vi "Reload Bitfile.vi"(8 "error in (no error)":errorcluster, 10 "RIO Addresses (all)":string[](array[string]), 11 "Node Ptr":u64) -> (0 "error out":errorcluster, 3 "Node Ptr out":T1=18446744073709551615 format="%.0x")   [LabVIEW 2015, in "Engine Simulation Toolkit System Explorer.lvlib"]
uses:
  Engine Simulation Toolkit System Explorer.lvlib
  <vilib>/NI Veristand/Custom Device API/Custom Device Item Ref.ctl
  Shared/Properties.vi
  <vilib>/NI Veristand/Custom Device API/Get Item Property (String Array).vi
  <vilib>/NI Veristand/Custom Device API/Get Item Property (Dependent File).vi
  <vilib>/NI VeriStand/Custom Device API/Custom Device API.lvlib
  Shared/Engine Simulation Toolkit Shared.lvlib
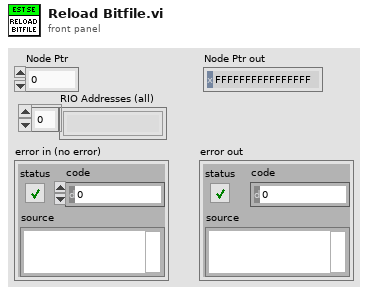
[diagram p1: front panel]
types:
  T1 = typedef "Custom Device API.lvlib/Custom Device Item Ref.ctl" = u64
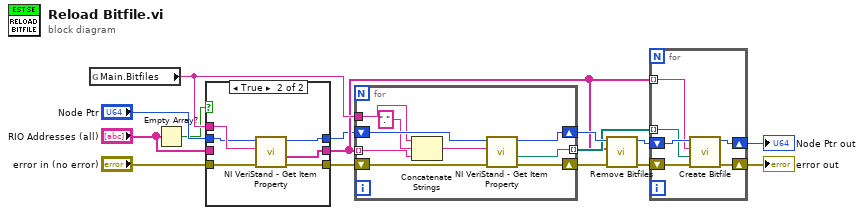
[diagram p0: block diagram]
diagram:
  n1 = global read "Properties.vi" "Main.Bitfiles"() -> (w15:string)
  n2 = Empty Array?(array="RIO Addresses (all)") -> (empty?=w2:bool)
  n3 = case shown="True" w2 {
    tunnel: w15 -> [_ w24]
    tunnel: [w18 w23] -> w11
    tunnel: [w17 w22] -> w10
    tunnel: [w16 w21] -> w9
    tunnel: "error in (no error)" -> [w17 w20]
    tunnel: "Node Ptr" -> [w16 w19]
    tunnel: "RIO Addresses (all)" -> [w18 _]
    frame False {
    }
    frame True {
      n4 = call-poly <vilib>:"NI VeriStand - Get Item Property.vi"("error in (no error)"=w20, "Property Name"=w24, "Item Ref in"=w19) -> ("error out"=w22:errorcluster, "Value"=w23:string[], "Item Ref out"=w21:T1)  [unwired: 5 in, 1 out]
    }
  }
  n5 = for {
    shift-right: [w30] -> w14
    shift-left: w9 -> [w33]
    shift-right: [w31] -> w13
    shift-left: w10 -> [w32]
    tunnel: w11 -> [w28] mode=indexing
    tunnel: [w26] -> w12 mode=indexing
    tunnel: w15 -> [w25]
    n6 = Concatenate Strings(w25, "." ("string"), w28) -> (w27:string)
    n7 = call-poly <vilib>:"NI VeriStand - Get Item Property.vi"("error in (no error)"=w32, "Property Name"=w27, "Item Ref in"=w33) -> ("error out"=w31:errorcluster, "Path"=w26:path, "Item Ref out"=w30:T1)  [unwired: 4 in, 2 out]
  }
  n8 = call "Remove Bitfiles.vi"("error in (no error)"=w13, "RIO Addresses"=w11, "Item Ref in"=w14) -> ("error out"=w4:errorcluster, "Item Ref out"=w8:T1)  [unwired: 5 in, 2 out]
  n9 = for {
    shift-right: [w38] -> w5
    shift-left: w4 -> [w39]
    shift-right: [w36] -> w3
    shift-left: w8 -> [w37]
    tunnel: w11 -> [w35] mode=indexing
    tunnel: w12 -> [w34] mode=indexing
    n10 = call "Create Bitfile.vi"("error in (no error)"=w39, "Bitfile Path in"=w34, "RIO Device Address in"=w35, "Item Ref in"=w37) -> ("error out"=w38:errorcluster, "Item Ref out"=w36:T1)  [unwired: 6 in]
  }
  "error out" <- w5
  "Node Ptr out" <- w3
